vi "_Number Count Down(Array).vi"(0 "fixed size array":i32[](array[numeric]), 1 "reset(F)":bool, 2 "threashold":i64=1000, 3 "Valid?(T)":bool) -> (6 "reach?":bool, 9 "left":i64[](array[numeric]))   [LabVIEW 2017]
uses:
  9de0e42d-c65c-4cbc-a92d-661ac054e2ac.vi
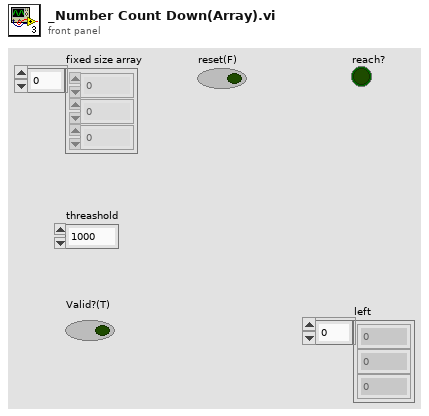
[diagram p1: front panel]
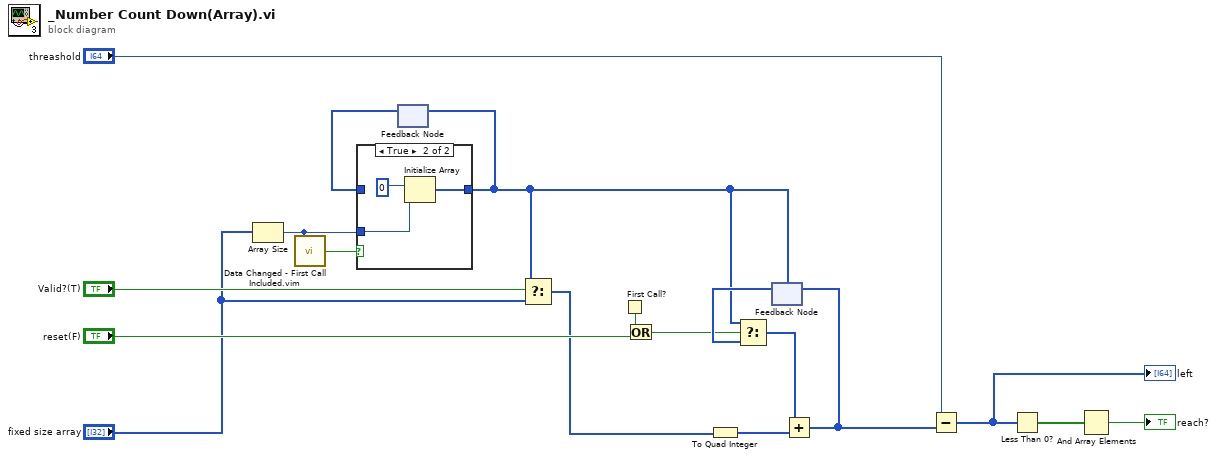
[diagram p0: block diagram]
diagram:
  n1 = Array Size(array="fixed size array") -> (size(s)=w5:i32)
  n2 = call "Data Changed - First Call Included.vim"("Variant"=w5) -> ("Changed"=w4:bool)
  n3 = feedback #1() -> (w2:i64[])  [unwired: 1 in]
  n4 = case shown="True" w4 {
    tunnel: w5 -> [_ w21]
    tunnel: [w19 w20] -> w3
    tunnel: w2 -> [w19 _]
    frame False {
    }
    frame True {
      n5 = Initialize Array(i64 0 ("threashold 2"), w21) -> (w20:i64[])
    }
  }
  n6 = feedback-in #1(w3) -> ()
  n7 = Select(t=w3, s="Valid?(T)", f="fixed size array") -> (s? t:f=w7:i64[])
  n8 = First Call?() -> (First Call?: T/F=w14:bool)
  n9 = Or(x=w14, y="reset(F)") -> (x .or. y?=w13:bool)
  n10 = To Quad Integer(1:w7) -> (0:w9:i64[])
  n11 = feedback #2(w3) -> (w18:i64[])
  n12 = Select(t=w3, s=w13, f=w18) -> (s? t:f=w15:i64[])
  n13 = Add(x=w15, y=w9) -> (x+y=w16:i64[])
  n14 = feedback-in #2(w16) -> ()
  n15 = Subtract(x="threashold", y=w16) -> (x-y=w11:i64[])
  "left" <- w11
  n16 = Less Than 0?(x=w11) -> (x < 0?=w10:bool[])
  n17 = And Array Elements(Boolean array=w10) -> (logical AND=→"reach?":bool)
